vi "RangeSearch.vi"(10 "Particle Report":T2, 11 "Particle Reports (Pixels)":T1(array[cluster])) -> (3 "배열":T1(array[cluster]))   [LabVIEW 2014]
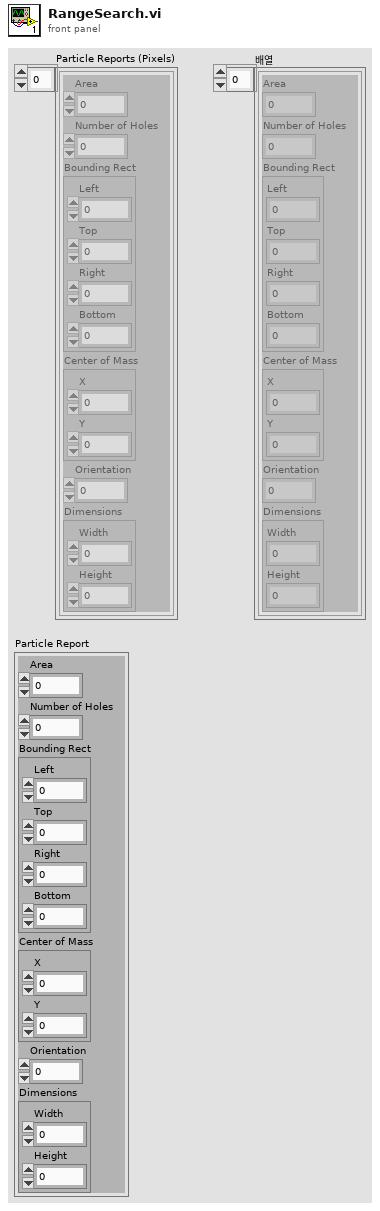
[diagram p1: front panel]
types:
  T1 = cluster{"Area":dbl, "Number of Holes":dbl, "Bounding Rect":cluster{"Left":dbl, "Top":dbl, "Right":dbl, "Bottom":dbl}, "Center of Mass":cluster{"X":dbl, "Y":dbl}, "Orientation":dbl, "Dimensions":cluster{"Width":dbl, "Height":dbl}}[]
  T2 = cluster{"Area":dbl, "Number of Holes":dbl, "Bounding Rect":cluster{"Left":dbl, "Top":dbl, "Right":dbl, "Bottom":dbl}, "Center of Mass":cluster{"X":dbl, "Y":dbl}, "Orientation":dbl, "Dimensions":cluster{"Width":dbl, "Height":dbl}}
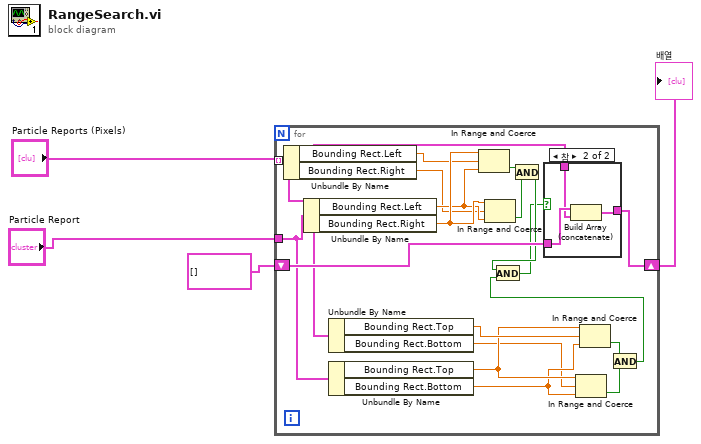
[diagram p0: block diagram]
diagram:
  n1 = for {
    tunnel: "Particle Reports (Pixels)" -> [w14] mode=indexing
    tunnel: "Particle Report" -> [w15]
    shift-right: [w23] -> w4
    shift-left: T1 [] -> [w22]
    n2 = Unbundle By Name(w14) -> ("Bounding Rect.Left"=w19:dbl, "Bounding Rect.Right"=w18:dbl)
    n3 = Unbundle By Name(w15) -> ("Bounding Rect.Left"=w20:dbl, "Bounding Rect.Right"=w21:dbl)
    n4 = Unbundle By Name(w14) -> ("Bounding Rect.Top"=w8:dbl, "Bounding Rect.Bottom"=w5:dbl)
    n5 = Unbundle By Name(w15) -> ("Bounding Rect.Top"=w7:dbl, "Bounding Rect.Bottom"=w6:dbl)
    n6 = In Range and Coerce(upper limit=w21, x=w19, lower limit=w20) -> (In Range?=w16:bool)  [unwired: 1 out]
    n7 = In Range and Coerce(upper limit=w21, x=w18, lower limit=w20) -> (In Range?=w17:bool)  [unwired: 1 out]
    n8 = And(x=w16, y=w17) -> (x .and. y?=w11:bool)
    n9 = In Range and Coerce(upper limit=w7, x=w5, lower limit=w6) -> (In Range?=w12:bool)  [unwired: 1 out]
    n10 = In Range and Coerce(upper limit=w7, x=w8, lower limit=w6) -> (In Range?=w13:bool)  [unwired: 1 out]
    n11 = And(x=w13, y=w12) -> (x .and. y?=w10:bool)
    n12 = And(x=w11, y=w10) -> (x .and. y?=w9:bool)
    n13 = case shown="참" w9 {
      tunnel: [w24 w27] -> w23
      tunnel: w22 -> [w24 w26]
      tunnel: w14 -> [_ w25]
      frame False {
      }
      frame True {
        n14 = Build Array (concatenate)(w26, w25) -> (w27:T1)
      }
    }
  }
  "배열" <- w4
